vi "Finish.vi"(4 "error in":errorcluster) -> ()   [LabVIEW 2013]
doc: "This VI is called just before exiting. It is expected to close I/O refnum, save collected data, etc."
uses:
  <vilib>/Rock Robotics/WPI/RobotDrive/WPI_RobotDriveGetSetRefNum.vi
  <vilib>/Rock Robotics/WPI/Joystick/WPI_JoystickGetSetRefNum.vi
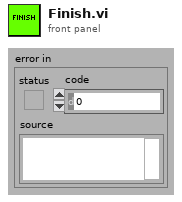
[diagram p1: front panel]
types:
  T1 = typedef "WPI_DigitalInputDevRef.ctl" = cluster{"DevStatus":errorcluster, "DIO Channel":T2, "Digital Module":T3}
  T2 = typedef "FPGA_DIOChannel.ctl" = enum8{"DIO 1", "DIO 2", "DIO 3", "DIO 4", "DIO 5", "DIO 6", "DIO 7", "DIO 8", "DIO 9", "DIO 10", "DIO 11", "DIO 12", "DIO 13", "DIO 14", "Invalid"}
  T3 = typedef "FPGA_TypedefDigitalModule.ctl" = enum16{"Digital Module 1", "Digital Module 2"}
  T4 = typedef "WPI_JoystickDevRef.ctl" = cluster{"Device":T5}
  T5 = typedef "WPI_JoystickDeviceEnum.ctl" = enum16{"USB 1", "USB 2", "USB 3", "USB 4", "Kinect 1", "Kinect 2"}
  T6 = typedef "WPI_CameraDevRef.ctl" = cluster{"Camera Address":string, "CameraStatus":errorcluster, "Acquire Image Notifier":refnum<notifier>}
  T7 = typedef "WPI_RobotDriveDevRef.ctl" = cluster{"DevStatus":errorcluster, "Motors[]":T8[], "Square Inputs":bool, "Max Output":dbl, "Isochronous":bool}
  T8 = typedef "WPI_MotorControlDeviceRef.ctl" = cluster{"DeviceStatus":errorcluster, "Type":enum16{"PWM", "CAN"}, "PWM":cluster{"Digital Module":T3, "PWM Channel":T9, "DeadBand":T10}, "CAN":cluster{"Device Number":u8, "Control Mode":T11, "Semaphore":T12, "Max Vout":dbl}, "Invert":bool, "TransformRef":T13, "InvTransformRef":T13}
  T9 = typedef "FPGA_DIOPWMChannel.ctl" = enum8{"PWM 1", "PWM 2", "PWM 3", "PWM 4", "PWM 5", "PWM 6", "PWM 7", "PWM 8", "PWM 9", "PWM 10", "Invalid"}
  T10 = typedef "WPI_PWMDeadband.ctl" = cluster{"Name":string, "maxPositivePwm":i32, "minPositivePwm":i32, "centerPwm":i32, "maxNegativePwm":i32, "minNegativePwm":i32, "angularRange":u16}
  T11 = typedef "WPI_CANJaguar_ControlMode.ctl" = enum8{"Percent VBus", "Current", "Speed", "Position", "Voltage"}
  T12 = typedef "Semaphore RefNum" = refnum<k1>
  T13 = typedef "WPI_PWMTransform_ConPane.ctl" = refnum<vi>
  T14 = typedef "WPI_EncoderDevRef.ctl" = cluster{"DevStatus":errorcluster, "EncoderIndex":T15, "CounterIndex":T16, "DistancePerCount":dbl, "Decoding Type":T17}
  T15 = typedef "FPGA_EncoderIdx.ctl" = enum8{"Enc 0", "Enc 1", "Enc 2", "Enc 3", "Invalid"}
  T16 = typedef "FPGA_CounterCtrSystemIndex.ctl" = enum8{"Ctr 0", "Ctr 1", "Ctr 2", "Ctr 3", "Ctr 4", "Ctr 5", "Ctr 6", "Ctr 7", "Invalid"}
  T17 = typedef "WPI_EncoderType.ctl" = enum16{"1x", "2x", "4x"}
  T18 = typedef "WPI_SolenoidDevRef.ctl" = cluster{"DevStatus":errorcluster, "Solenoid Module":T19, "Forward Solenoid Channel":T20, "Reverse Solenoid Channel":T20}
  T19 = typedef "FPGA_TypedefSolenoidModule.ctl" = enum16{"Solenoid Module 1", "Solenoid Module 2"}
  T20 = typedef "WPI_SolenoidChannel.ctl" = enum8{"Solenoid 1", "Solenoid 2", "Solenoid 3", "Solenoid 4", "Solenoid 5", "Solenoid 6", "Solenoid 7", "Solenoid 8", "Invalid"}
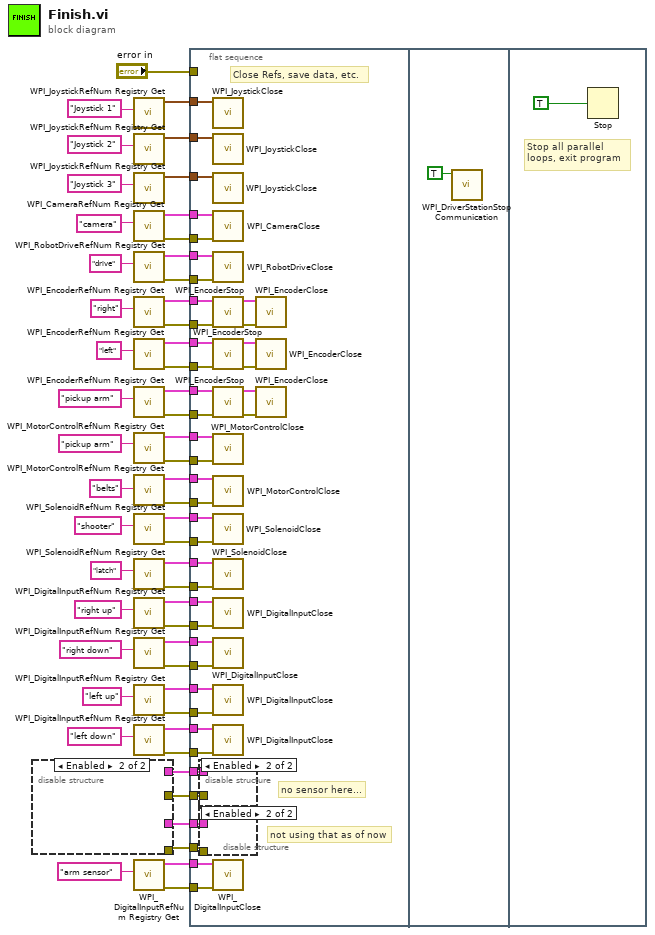
[diagram p0: block diagram]
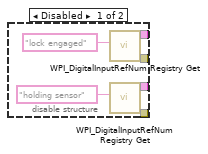
[diagram p2: hidden frame]
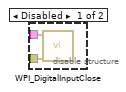
[diagram p3: hidden frame]
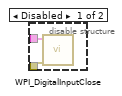
[diagram p4: hidden frame]
diagram:
  n1 = disable-structure shown="Enabled" {
    disable-tunnel: [w59 _] -> w5
    disable-tunnel: [w58 _] -> w4
    disable-tunnel: [w56 _] -> w2
    disable-tunnel: [w55 _] -> w1
    frame Disabled {
      n2 = call <vilib>:"WPI_DigitalInputRefNum Registry Get.vi"("refnum name"="lock engaged") -> ("error out"=w56:errorcluster, "DigitalInputDevRef"=w55:T1)  [unwired: 9 in]
      n3 = call <vilib>:"WPI_DigitalInputRefNum Registry Get.vi"("refnum name"="holding sensor") -> ("error out"=w59:errorcluster, "DigitalInputDevRef"=w58:T1)  [unwired: 9 in]
    }
    frame Enabled {
    }
  }
  n4 = call <vilib>:"WPI_JoystickRefNum Registry Get.vi"("refnum name"="Joystick 1") -> ("JoystickDevRef"=w52:T4)  [unwired: 1 in, 9 out]
  n5 = call <vilib>:"WPI_JoystickRefNum Registry Get.vi"("refnum name"="Joystick 2") -> ("JoystickDevRef"=w49:T4)  [unwired: 1 in, 9 out]
  n6 = call <vilib>:"WPI_JoystickRefNum Registry Get.vi"("refnum name"="Joystick 3") -> ("JoystickDevRef"=w46:T4)  [unwired: 1 in, 9 out]
  n7 = call <vilib>:"WPI_CameraRefNum Registry Get.vi"("refnum name"="camera") -> ("error out"=w39:errorcluster, "CameraDevRef"=w51:T6)  [unwired: 1 in, 8 out]
  n8 = call <vilib>:"WPI_RobotDriveRefNum Registry Get.vi"("refnum name"="drive") -> ("error out"=w38:errorcluster, "RobotDriveDevRef"=w44:T7)  [unwired: 9 in]
  n9 = call <vilib>:"WPI_EncoderRefNum Registry Get.vi"("refnum name"="right") -> ("error out"=w37:errorcluster, "EncoderDevRef"=w41:T14)  [unwired: 9 in]
  n10 = call <vilib>:"WPI_EncoderRefNum Registry Get.vi"("refnum name"="left") -> ("error out"=w36:errorcluster, "EncoderDevRef"=w40:T14)  [unwired: 9 in]
  n11 = call <vilib>:"WPI_EncoderRefNum Registry Get.vi"("refnum name"="pickup arm") -> ("error out"=w35:errorcluster, "EncoderDevRef"=w33:T14)  [unwired: 9 in]
  n12 = call <vilib>:"WPI_MotorControlRefNum Registry Get.vi"("refnum name"="pickup arm") -> ("error out"=w29:errorcluster, "MotorControlDevRef"=w30:T8)  [unwired: 9 in]
  n13 = call <vilib>:"WPI_MotorControlRefNum Registry Get.vi"("refnum name"="belts") -> ("error out"=w27:errorcluster, "MotorControlDevRef"=w28:T8)  [unwired: 9 in]
  n14 = call <vilib>:"WPI_SolenoidRefNum Registry Get.vi"("refnum name"="shooter") -> ("error out"=w25:errorcluster, "SolenoidDevRef"=w26:T18)  [unwired: 9 in]
  n15 = call <vilib>:"WPI_SolenoidRefNum Registry Get.vi"("refnum name"="latch") -> ("error out"=w21:errorcluster, "SolenoidDevRef"=w22:T18)  [unwired: 9 in]
  n16 = call <vilib>:"WPI_DigitalInputRefNum Registry Get.vi"("refnum name"="right up") -> ("error out"=w14:errorcluster, "DigitalInputDevRef"=w15:T1)  [unwired: 9 in]
  n17 = call <vilib>:"WPI_DigitalInputRefNum Registry Get.vi"("refnum name"="right down") -> ("error out"=w12:errorcluster, "DigitalInputDevRef"=w13:T1)  [unwired: 9 in]
  n18 = call <vilib>:"WPI_DigitalInputRefNum Registry Get.vi"("refnum name"="left up") -> ("error out"=w10:errorcluster, "DigitalInputDevRef"=w11:T1)  [unwired: 9 in]
  n19 = call <vilib>:"WPI_DigitalInputRefNum Registry Get.vi"("refnum name"="left down") -> ("error out"=w8:errorcluster, "DigitalInputDevRef"=w9:T1)  [unwired: 9 in]
  n20 = call <vilib>:"WPI_DigitalInputRefNum Registry Get.vi"("refnum name"="arm sensor") -> ("error out"=w7:errorcluster, "DigitalInputDevRef"=w6:T1)  [unwired: 9 in]
  n21 = flat-sequence {
    tunnel: w52 -> [w100]
    tunnel: w51 -> [w99]
    tunnel: w49 -> [w98]
    tunnel: w46 -> [w97]
    tunnel: w44 -> [w96]
    tunnel: w41 -> [w95]
    tunnel: w40 -> [w88]
    tunnel: w39 -> [w92]
    tunnel: w38 -> [w91]
    tunnel: w37 -> [w90]
    tunnel: w36 -> [w89]
    tunnel: w35 -> [w84]
    tunnel: w33 -> [w83]
    tunnel: w30 -> [w81]
    tunnel: w29 -> [w80]
    tunnel: w28 -> [w78]
    tunnel: w27 -> [w79]
    tunnel: w26 -> [w76]
    tunnel: w25 -> [w77]
    tunnel: w22 -> [w74]
    tunnel: w21 -> [w75]
    tunnel: "error in" -> [_]
    tunnel: w15 -> [w69]
    tunnel: w14 -> [w70]
    tunnel: w13 -> [w68]
    tunnel: w12 -> [w71]
    tunnel: w11 -> [w67]
    tunnel: w10 -> [w72]
    tunnel: w9 -> [w66]
    tunnel: w8 -> [w73]
    tunnel: w4 -> [w64]
    tunnel: w5 -> [w63]
    tunnel: w6 -> [w65]
    tunnel: w7 -> [w62]
    tunnel: w1 -> [w61]
    tunnel: w2 -> [w60]
    frame #0 {
      # "no sensor here..."
      # "not using that as of now"
      # "Close Refs, save data, etc."
      n22 = disable-structure shown="Enabled" {
        disable-tunnel: w61 -> [w102 _]
        disable-tunnel: w60 -> [w101 _]
        frame Disabled {
          n23 = call <vilib>:"WPI_DigitalInputClose.vi"("error in (no error)"=w101, "DigitalInputDevRef"=w102) -> ()  [unwired: 9 in, 1 out]
        }
        frame Enabled {
        }
      }
      n24 = disable-structure shown="Enabled" {
        disable-tunnel: w64 -> [w104 _]
        disable-tunnel: w63 -> [w103 _]
        frame Disabled {
          n25 = call <vilib>:"WPI_DigitalInputClose.vi"("error in (no error)"=w103, "DigitalInputDevRef"=w104) -> ()  [unwired: 9 in, 1 out]
        }
        frame Enabled {
        }
      }
      n26 = call <vilib>:"WPI_JoystickClose.vi"("JoystickDevRef"=w100) -> ()  [unwired: 11 out]
      n27 = call <vilib>:"WPI_JoystickClose.vi"("JoystickDevRef"=w98) -> ()  [unwired: 11 out]
      n28 = call <vilib>:"WPI_JoystickClose.vi"("JoystickDevRef"=w97) -> ()  [unwired: 11 out]
      n29 = call <vilib>:"WPI_CameraClose.vi"("error in (no error)"=w92, "CameraDevRef"=w99) -> ()  [unwired: 10 out]
      n30 = call <vilib>:"WPI_RobotDriveClose.vi"("error in (no error)"=w91, "RobotDriveDevRef"=w96) -> ()  [unwired: 9 in, 1 out]
      n31 = call <vilib>:"WPI_EncoderStop.vi"("error in (no error)"=w90, "EncoderDevRef"=w95) -> ("error out"=w94:errorcluster, "EncoderDevRef"=w93:T14)  [unwired: 8 in]
      n32 = call <vilib>:"WPI_EncoderStop.vi"("error in (no error)"=w89, "EncoderDevRef"=w88) -> ("error out"=w86:errorcluster, "EncoderDevRef"=w87:T14)  [unwired: 8 in]
      n33 = call <vilib>:"WPI_EncoderStop.vi"("error in (no error)"=w84, "EncoderDevRef"=w83) -> ("error out"=w85:errorcluster, "EncoderDevRef"=w82:T14)  [unwired: 8 in]
      n34 = call <vilib>:"WPI_MotorControlClose.vi"("error in (no error)"=w80, "MotorControlDevRef"=w81) -> ()  [unwired: 9 in, 1 out]
      n35 = call <vilib>:"WPI_MotorControlClose.vi"("error in (no error)"=w79, "MotorControlDevRef"=w78) -> ()  [unwired: 9 in, 1 out]
      n36 = call <vilib>:"WPI_SolenoidClose.vi"("error in (no error)"=w77, "SolenoidDevRef"=w76) -> ()  [unwired: 9 in, 1 out]
      n37 = call <vilib>:"WPI_SolenoidClose.vi"("error in (no error)"=w75, "SolenoidDevRef"=w74) -> ()  [unwired: 9 in, 1 out]
      n38 = call <vilib>:"WPI_DigitalInputClose.vi"("error in (no error)"=w70, "DigitalInputDevRef"=w69) -> ()  [unwired: 9 in, 1 out]
      n39 = call <vilib>:"WPI_DigitalInputClose.vi"("error in (no error)"=w71, "DigitalInputDevRef"=w68) -> ()  [unwired: 9 in, 1 out]
      n40 = call <vilib>:"WPI_DigitalInputClose.vi"("error in (no error)"=w72, "DigitalInputDevRef"=w67) -> ()  [unwired: 9 in, 1 out]
      n41 = call <vilib>:"WPI_DigitalInputClose.vi"("error in (no error)"=w73, "DigitalInputDevRef"=w66) -> ()  [unwired: 9 in, 1 out]
      n42 = call <vilib>:"WPI_DigitalInputClose.vi"("error in (no error)"=w62, "DigitalInputDevRef"=w65) -> ()  [unwired: 9 in, 1 out]
      n43 = call <vilib>:"WPI_EncoderClose.vi"("error in (no error)"=w94, "EncoderDevRef"=w93) -> ()  [unwired: 9 in, 1 out]
      n44 = call <vilib>:"WPI_EncoderClose.vi"("error in (no error)"=w86, "EncoderDevRef"=w87) -> ()  [unwired: 9 in, 1 out]
      n45 = call <vilib>:"WPI_EncoderClose.vi"("error in (no error)"=w85, "EncoderDevRef"=w82) -> ()  [unwired: 9 in, 1 out]
    }
    frame #1 {
      n46 = call <vilib>:"WPI_DriverStationStop Communication.vi"("StopCommunication"=TRUE) -> ()  [unwired: 10 in, 1 out]
    }
    frame #2 {
      # "Stop all parallel\nloops, exit program"
      n47 = Stop(stop? (T)=TRUE ("Quit")) -> ()
    }
  }
